vi "Day 8.vi"() -> ()   [LabVIEW 2021]
uses:
  b2847cdb-c60e-4571-aa0a-510e0b01ddce.vi
  7a7e40d0-1107-41e4-9caf-784d51971341.vi
  52a580fe-a730-4ecf-827f-bdb76e2bd2ae.vi
  2b776e78-9b69-4ed1-853f-875d71f7d19c.vi
  6051aadd-e33c-4c9e-8f10-c58bb75e1c96.vi
  c10b95b6-e31f-4627-b78a-c608f1f96919.vi
  <vilib>/Utility/file.llb/Read Delimited Spreadsheet (string).vi
panel:
  out "Input":string[][](array[string])
  out "Solution":i64
  in  "Input File":enum32{"example input", "input"}(radio)
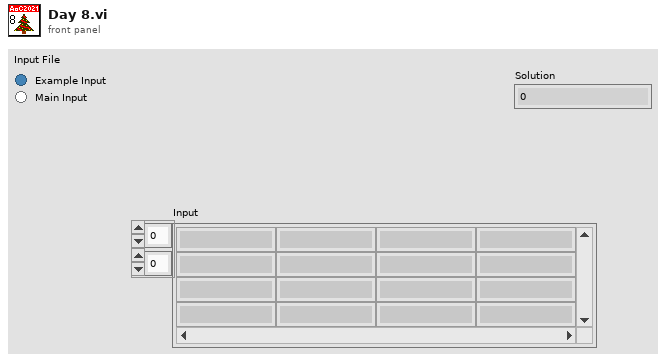
[diagram p1: front panel]
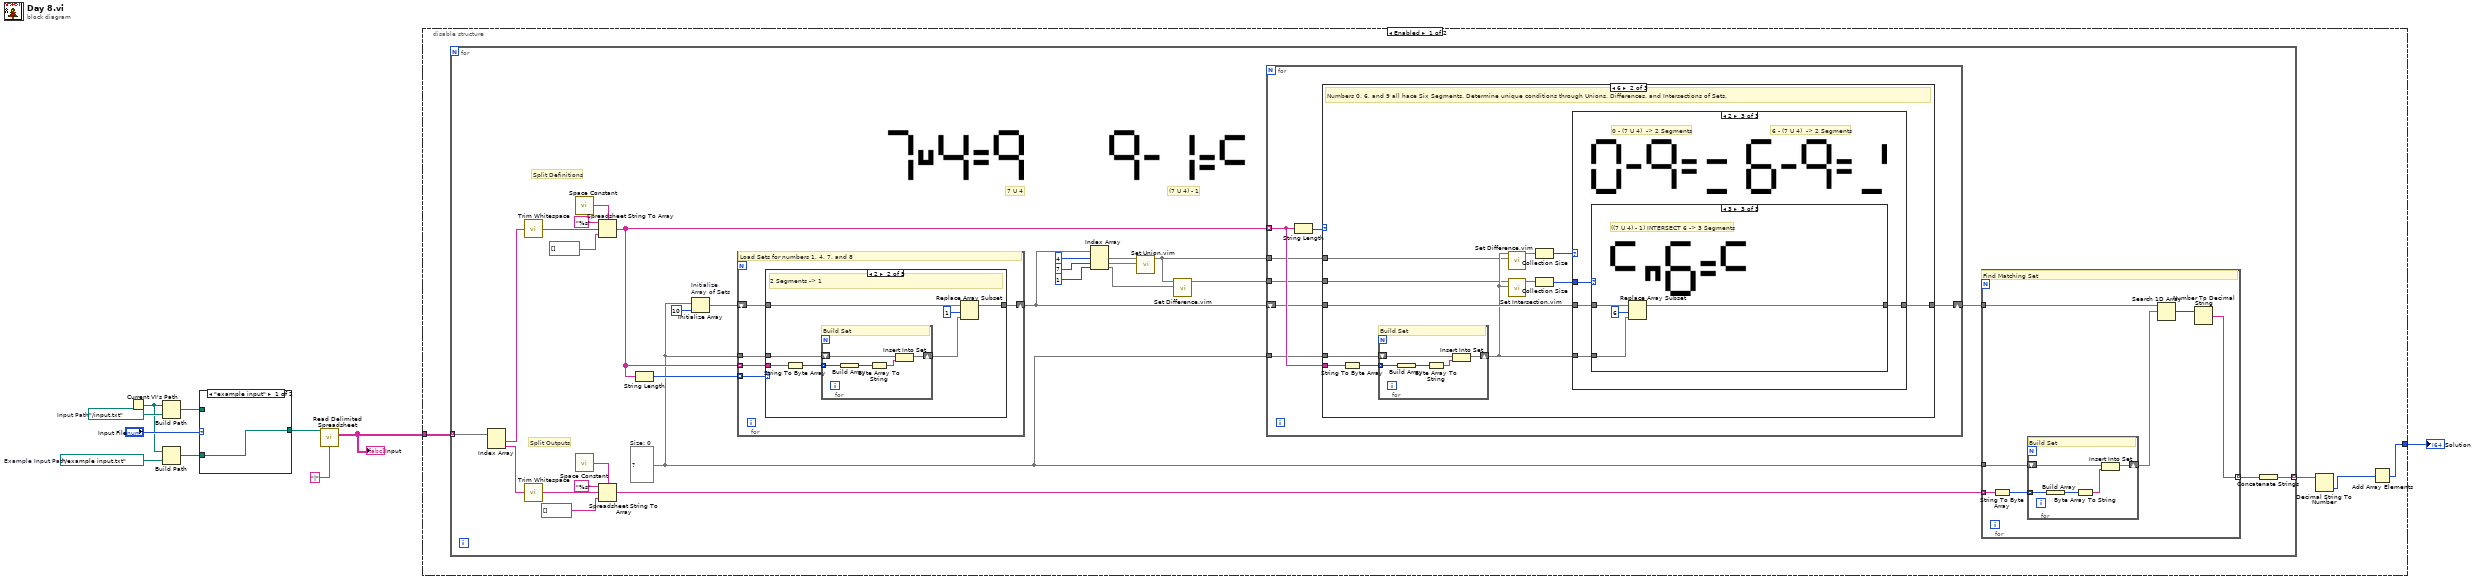
[diagram p0: block diagram]
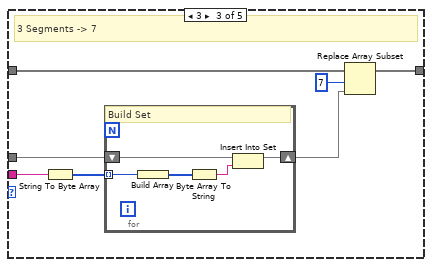
[diagram p3: hidden frame]
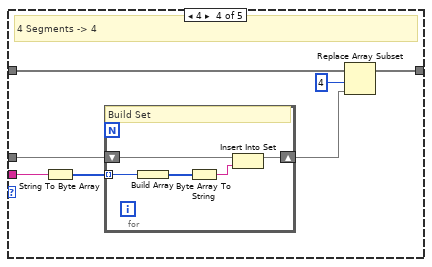
[diagram p4: hidden frame]
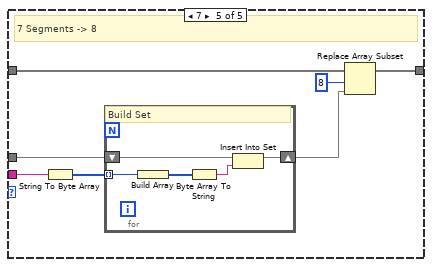
[diagram p5: hidden frame]
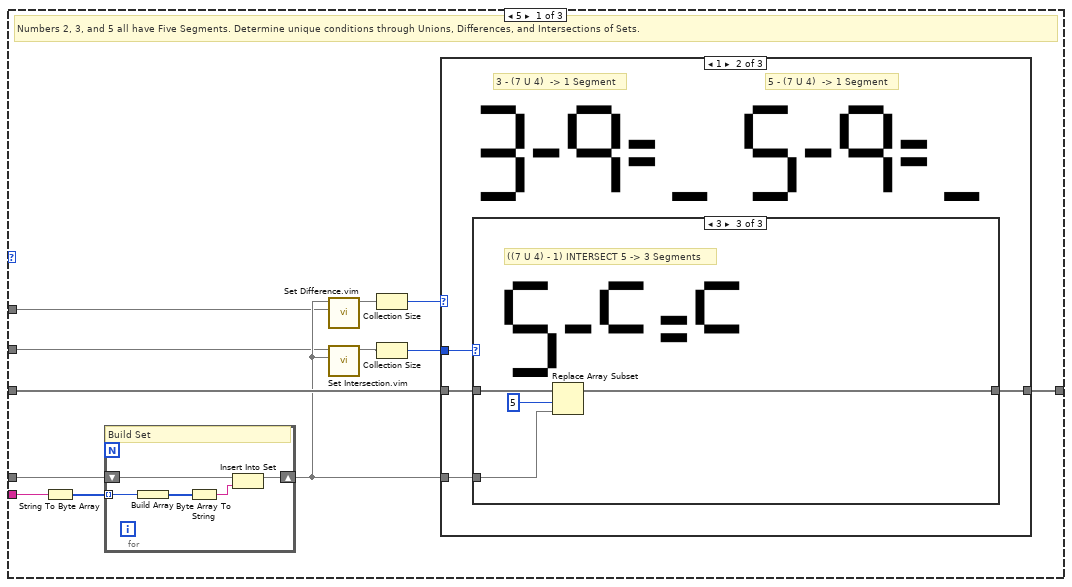
[diagram p6: hidden frame]
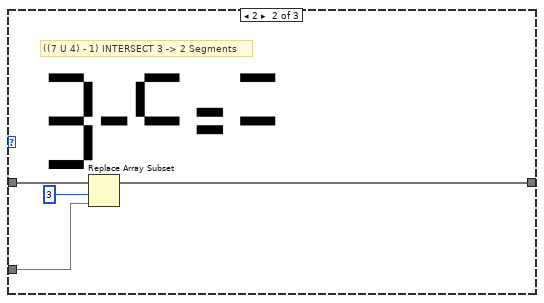
[diagram p9: hidden frame]
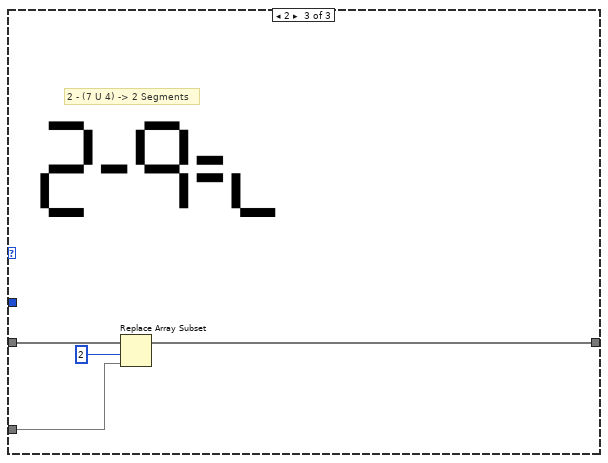
[diagram p10: hidden frame]
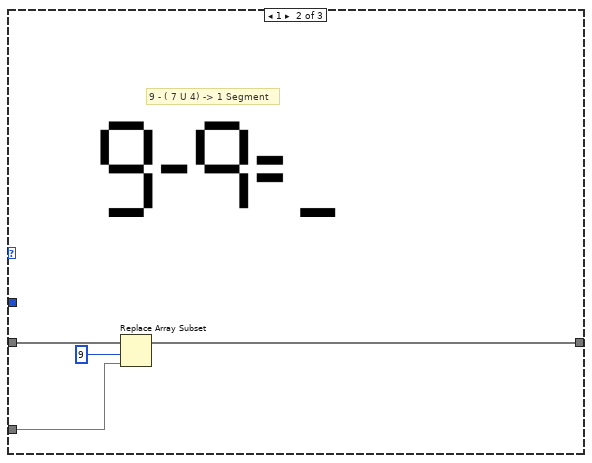
[diagram p12: hidden frame]
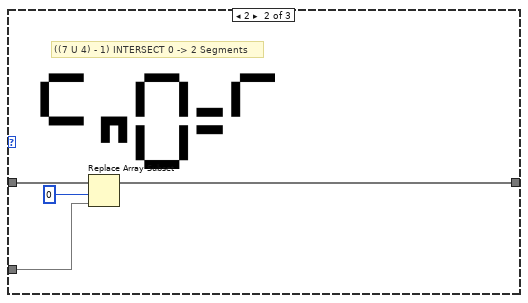
[diagram p14: hidden frame]
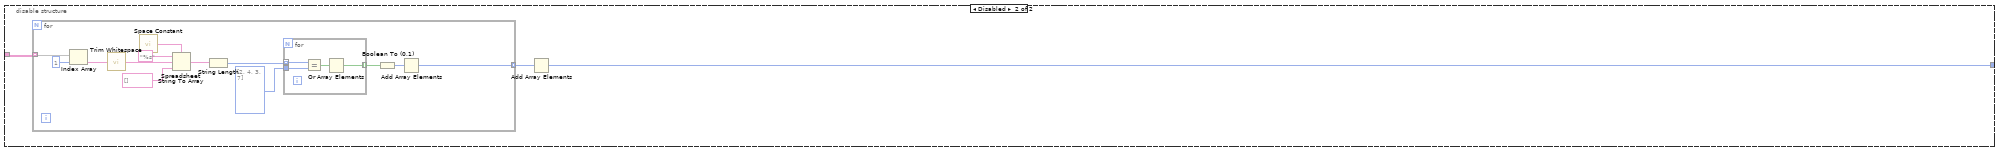
[diagram p16: hidden frame]
diagram:
  w9 = path "../example input.txt"  # Example Input Path
  w10 = path "../input.txt"  # Input Path
  n1 = Current VI's Path() -> (path=w4:path)
  n2 = Build Path(base path=w4, name or relative path=w10) -> (appended path=w7:path)
  n3 = Build Path(base path=w4, name or relative path=w9) -> (appended path=w6:path)
  n4 = case shown="\"example input\"" "Input File" {
    tunnel: w7 -> [_ w12]
    tunnel: w6 -> [w11 _]
    tunnel: [w11 w12] -> w5
    frame "example input" {
    }
    frame "input" {
    }
  }
  n5 = call-poly <vilib>:"Read Delimited Spreadsheet.vi"("file path (dialog if empty)"=w5, "delimiter (\\t)"="|" ("delimiter (\\t)")) -> ("all rows"=w1:string[][])  [unwired: 8 in, 5 out]
  "Input" <- w1
  n6 = disable-structure shown="Enabled" {
    disable-tunnel: w1 -> [w16 w192]
    disable-tunnel: [w15 w190] -> w3
    frame Enabled {
      n7 = for {
        tunnel: w16 -> [w44] mode=indexing
        tunnel: [w39] -> w14 mode=indexing
        w26 = set{string} {}  # Size: 0
        # "(7 U 4) - 1"
        # "7 U 4"
        # "Split Outputs"
        # "Split Definitions"
        n8 = Index Array(array=w44) -> (element #1=w34:string, element #2=w45:string)  [unwired: 2 in]
        n9 = call <vilib>:"Trim Whitespace.vi"("string"=w34) -> ("trimmed string"=w35:string)  [unwired: 1 in]
        n10 = call <vilib>:"Trim Whitespace.vi"("string"=w45) -> ("trimmed string"=w43:string)  [unwired: 1 in]
        n11 = call <vilib>:"Space Constant.vi"() -> ("String"=w38:string)
        n12 = call <vilib>:"Space Constant.vi"() -> ("String"=w40:string)
        n13 = Spreadsheet String To Array(delimiter (Tab)=w38, format string="%s", spreadsheet string=w35, array type (2D Dbl)=string[] []) -> (array=w30:string[])
        n14 = Spreadsheet String To Array(delimiter (Tab)=w40, format string="%s", spreadsheet string=w43, array type (2D Dbl)=string[] []) -> (array=w33:string[])
        n15 = String Length(string=w30) -> (length=w31:i32[])
        n16 = Initialize Array "Initialize\nArray of Sets"(w26, 10 ("dimension size")) -> (w28:set{string}[])
        n17 = for {
          tunnel: w31 -> [w50] mode=indexing
          tunnel: w30 -> [w49] mode=indexing
          shift-right: [w46] -> w19
          shift-left: w28 -> [w48]
          tunnel: w26 -> [w47]
          # "Load Sets for numbers 1, 4, 7, and 8"
          n18 = case shown="2" w50 {
            tunnel: w49 -> [_ w58 w70 w82 w94]
            tunnel: w48 -> [w51 w55 w67 w79 w91]
            tunnel: w47 -> [_ w56 w68 w80 w92]
            tunnel: [w51 w52 w64 w76 w88] -> w46
            frame 0, Default {
            }
            frame 2 {
              # "2 Segments -> 1"
              n19 = String To Byte Array(string=w58) -> (unsigned byte array=w57:u8[])
              n20 = for {
                tunnel: w57 -> [w63] mode=indexing
                shift-right: [w60] -> w54
                shift-left: w56 -> [w59]
                # "Build Set"
                n21 = Build Array(w63) -> (w61:u8[])
                n22 = Byte Array To String(unsigned byte array=w61) -> (string=w62:string)
                n23 = Insert Into Set(10:w62, 11:w59) -> (3:w60:set{string})  [unwired: 1 out]
              }
              n24 = Replace Array Subset(array=w55, new element=w54, index=1) -> (w52:set{string}[])
            }
            frame 3 {
              # "3 Segments -> 7"
              n25 = String To Byte Array(string=w70) -> (unsigned byte array=w69:u8[])
              n26 = for {
                tunnel: w69 -> [w75] mode=indexing
                shift-right: [w72] -> w66
                shift-left: w68 -> [w71]
                # "Build Set"
                n27 = Build Array(w75) -> (w73:u8[])
                n28 = Byte Array To String(unsigned byte array=w73) -> (string=w74:string)
                n29 = Insert Into Set(10:w74, 11:w71) -> (3:w72:set{string})  [unwired: 1 out]
              }
              n30 = Replace Array Subset(array=w67, new element=w66, index=7) -> (w64:set{string}[])
            }
            frame 4 {
              # "4 Segments -> 4"
              n31 = String To Byte Array(string=w82) -> (unsigned byte array=w81:u8[])
              n32 = for {
                tunnel: w81 -> [w87] mode=indexing
                shift-right: [w84] -> w78
                shift-left: w80 -> [w83]
                # "Build Set"
                n33 = Build Array(w87) -> (w85:u8[])
                n34 = Byte Array To String(unsigned byte array=w85) -> (string=w86:string)
                n35 = Insert Into Set(10:w86, 11:w83) -> (3:w84:set{string})  [unwired: 1 out]
              }
              n36 = Replace Array Subset(array=w79, new element=w78, index=4) -> (w76:set{string}[])
            }
            frame 7 {
              # "7 Segments -> 8"
              n37 = String To Byte Array(string=w94) -> (unsigned byte array=w93:u8[])
              n38 = for {
                tunnel: w93 -> [w99] mode=indexing
                shift-right: [w96] -> w90
                shift-left: w92 -> [w95]
                # "Build Set"
                n39 = Build Array(w99) -> (w97:u8[])
                n40 = Byte Array To String(unsigned byte array=w97) -> (string=w98:string)
                n41 = Insert Into Set(10:w98, 11:w95) -> (3:w96:set{string})  [unwired: 1 out]
              }
              n42 = Replace Array Subset(array=w91, new element=w90, index=8) -> (w88:set{string}[])
            }
          }
        }
        n43 = Index Array(array=w19, index #1=4 ("index"), index #2=7 ("index"), index #3=1 ("index")) -> (element #1=w22:set{string}, element #2=w23:set{string}, element #3=w25:set{string})
        n44 = call "Set Union.vim"("set 2"=w23, "set 1"=w22) -> ("union"=w18:set{string})  [unwired: 9 in]
        n45 = call "Set Difference.vim"("set 2"=w25, "set 1"=w18) -> ("difference"=w17:set{string})  [unwired: 9 in]
        n46 = for {
          tunnel: w30 -> [w105] mode=indexing
          tunnel: w26 -> [w104]
          shift-right: [w102] -> w27
          shift-left: w19 -> [w103]
          tunnel: w18 -> [w101]
          tunnel: w17 -> [w100]
          n47 = String Length(string=w105) -> (length=w106:i32)
          n48 = case shown="6" w106 {
            tunnel: w105 -> [w117 w152 _]
            tunnel: w104 -> [w116 w151 _]
            tunnel: w103 -> [w114 w149 w177]
            tunnel: [w113 w148 w177] -> w102
            tunnel: w101 -> [w108 w143 _]
            tunnel: w100 -> [w107 w142 _]
            frame 5 {
              # "Numbers 2, 3, and 5 all have Five Segments. Determine unique conditions through Unions, Differences, and Intersections of Sets."
              n49 = String To Byte Array(string=w117) -> (unsigned byte array=w118:u8[])
              n50 = for {
                tunnel: w118 -> [w123] mode=indexing
                shift-right: [w120] -> w110
                shift-left: w116 -> [w119]
                # "Build Set"
                n51 = Build Array(w123) -> (w121:u8[])
                n52 = Byte Array To String(unsigned byte array=w121) -> (string=w122:string)
                n53 = Insert Into Set(10:w122, 11:w119) -> (3:w120:set{string})  [unwired: 1 out]
              }
              n54 = call "Set Difference.vim"("set 2"=w108, "set 1"=w110) -> ("difference"=w112:set{string})  [unwired: 9 in]
              n55 = call "Set Intersection.vim"("set 2"=w110, "set 1"=w107) -> ("intersection"=w109:set{string})  [unwired: 9 in]
              n56 = Collection Size(1:w112) -> (0:w115:i32)
              n57 = Collection Size(1:w109) -> (0:w111:i32)
              n58 = case shown="1" w115 {
                tunnel: w110 -> [_ w126 w138]
                tunnel: w114 -> [w124 w128 w140]
                tunnel: [w124 w127 w139] -> w113
                tunnel: w111 -> [_ w125 _]
                frame 0, Default {
                }
                frame 1 {
                  # "5 - (7 U 4)  -> 1 Segment"
                  # "3 - (7 U 4)  -> 1 Segment"
                  n59 = case shown="3" w125 {
                    tunnel: w128 -> [w129 w132 w136]
                    tunnel: [w129 w131 w135] -> w127
                    tunnel: w126 -> [_ w130 w134]
                    frame Default {
                    }
                    frame 2 {
                      # "((7 U 4) - 1) INTERSECT 3 -> 2 Segments"
                      n60 = Replace Array Subset(array=w132, new element=w130, index=3) -> (w131:set{string}[])
                    }
                    frame 3 {
                      # "((7 U 4) - 1) INTERSECT 5 -> 3 Segments"
                      n61 = Replace Array Subset(array=w136, new element=w134, index=5) -> (w135:set{string}[])
                    }
                  }
                }
                frame 2 {
                  # "2 - (7 U 4) -> 2 Segments"
                  n62 = Replace Array Subset(array=w140, new element=w138, index=2) -> (w139:set{string}[])
                }
              }
            }
            frame 6 {
              # "Numbers 0, 6, and 9 all hace Six Segments. Determine unique conditions through Unions, Differences, and Intersections of Sets."
              n63 = String To Byte Array(string=w152) -> (unsigned byte array=w153:u8[])
              n64 = for {
                tunnel: w153 -> [w158] mode=indexing
                shift-right: [w155] -> w145
                shift-left: w151 -> [w154]
                # "Build Set"
                n65 = Build Array(w158) -> (w156:u8[])
                n66 = Byte Array To String(unsigned byte array=w156) -> (string=w157:string)
                n67 = Insert Into Set(10:w157, 11:w154) -> (3:w155:set{string})  [unwired: 1 out]
              }
              n68 = call "Set Difference.vim"("set 2"=w143, "set 1"=w145) -> ("difference"=w147:set{string})  [unwired: 9 in]
              n69 = call "Set Intersection.vim"("set 2"=w145, "set 1"=w142) -> ("intersection"=w144:set{string})  [unwired: 9 in]
              n70 = Collection Size(1:w147) -> (0:w150:i32)
              n71 = Collection Size(1:w144) -> (0:w146:i32)
              n72 = case shown="2" w150 {
                tunnel: w145 -> [_ w160 w165]
                tunnel: w149 -> [w159 w162 w167]
                tunnel: [w159 w161 w166] -> w148
                tunnel: w146 -> [_ _ w164]
                frame 0, Default {
                }
                frame 1 {
                  # "9 - ( 7 U 4) -> 1 Segment"
                  n73 = Replace Array Subset(array=w162, new element=w160, index=9) -> (w161:set{string}[])
                }
                frame 2 {
                  # "6 - (7 U 4)  -> 2 Segments"
                  # "0 - (7 U 4)  -> 2 Segments"
                  n74 = case shown="3" w164 {
                    tunnel: w167 -> [w168 w171 w175]
                    tunnel: [w168 w170 w174] -> w166
                    tunnel: w165 -> [_ w169 w173]
                    frame Default {
                    }
                    frame 2 {
                      # "((7 U 4) - 1) INTERSECT 0 -> 2 Segments"
                      n75 = Replace Array Subset(array=w171, new element=w169, index=0) -> (w170:set{string}[])
                    }
                    frame 3 {
                      # "((7 U 4) - 1) INTERSECT 6 -> 3 Segments"
                      n76 = Replace Array Subset(array=w175, new element=w173, index=6) -> (w174:set{string}[])
                    }
                  }
                }
              }
            }
            frame Default {
            }
          }
        }
        n77 = for {
          tunnel: w33 -> [w183] mode=indexing
          tunnel: [w178] -> w32 mode=indexing
          tunnel: w26 -> [w182]
          tunnel: w27 -> [w181]
          # "Find Matching Set"
          n78 = String To Byte Array(string=w183) -> (unsigned byte array=w184:u8[])
          n79 = for {
            tunnel: w184 -> [w189] mode=indexing
            shift-right: [w186] -> w180
            shift-left: w182 -> [w185]
            # "Build Set"
            n80 = Build Array(w189) -> (w187:u8[])
            n81 = Byte Array To String(unsigned byte array=w187) -> (string=w188:string)
            n82 = Insert Into Set(10:w188, 11:w185) -> (3:w186:set{string})  [unwired: 1 out]
          }
          n83 = Search 1D Array(1D array=w181, element=w180) -> (index of element=w179:i32)  [unwired: 1 in]
          n84 = Number To Decimal String(number=w179) -> (decimal integer string=w178:string)  [unwired: 1 in]
        }
        n85 = Concatenate Strings(w32) -> (w39:string)
      }
      n86 = Decimal String To Number(string=w14) -> (number=w13:i32[])  [unwired: 2 in, 1 out]
      n87 = Add Array Elements(numeric array=w13) -> (sum=w15:i32)
    }
    frame Disabled {
      n88 = for {
        tunnel: w192 -> [w203] mode=indexing
        tunnel: [w193] -> w191 mode=indexing
        n89 = Index Array(array=w203, index=1) -> (element=w204:string)
        n90 = call <vilib>:"Trim Whitespace.vi"("string"=w204) -> ("trimmed string"=w202:string)  [unwired: 1 in]
        n91 = call <vilib>:"Space Constant.vi"() -> ("String"=w199:string)
        n92 = Spreadsheet String To Array(delimiter (Tab)=w199, format string="%s", spreadsheet string=w202, array type (2D Dbl)=string[] []) -> (array=w198:string[])
        n93 = String Length(string=w198) -> (length=w197:i32[])
        n94 = for {
          tunnel: w197 -> [w209] mode=indexing
          tunnel: i32[] [2, 4, 3, 7] -> [w208]
          tunnel: [w206] -> w195 mode=indexing
          n95 = Equal?(x=w209, y=w208) -> (x = y?=w207:bool[])
          n96 = Or Array Elements(Boolean array=w207) -> (logical OR=w206:bool)
        }
        n97 = Boolean To (0,1)(Boolean=w195) -> (0, 1=w194:i16[])
        n98 = Add Array Elements(numeric array=w194) -> (sum=w193:i16)
      }
      n99 = Add Array Elements(numeric array=w191) -> (sum=w190:i16)
    }
  }
  "Solution" <- w3
